vi "Uart log catch.vi"() -> (10 "Key word 2":i32)   [LabVIEW 2023]
uses:
  <vilib>/Instr/_visa.llb/VISA Configure Serial Port (Instr).vi
  <vilib>/Utility/file.llb/Write Delimited Spreadsheet (string).vi
panel:
  in  "Combo Box 3":string(combo)="mfc"
  in  "Combo Box 2":string(combo)="nu1651"
  in  "search string":string="mfc_auto_test_work: g_auto_test_step = 0x"
  in  "Combo Box":string(combo)="mfc_auto_test_work"
  in  "Clear":bool
  in  "VISA resource name":refnum<visa-resource-name>="COM15"
  out "Key word log 2":string
  out "Key word log 1":string
  out "Full log":string
  in  "stop":bool
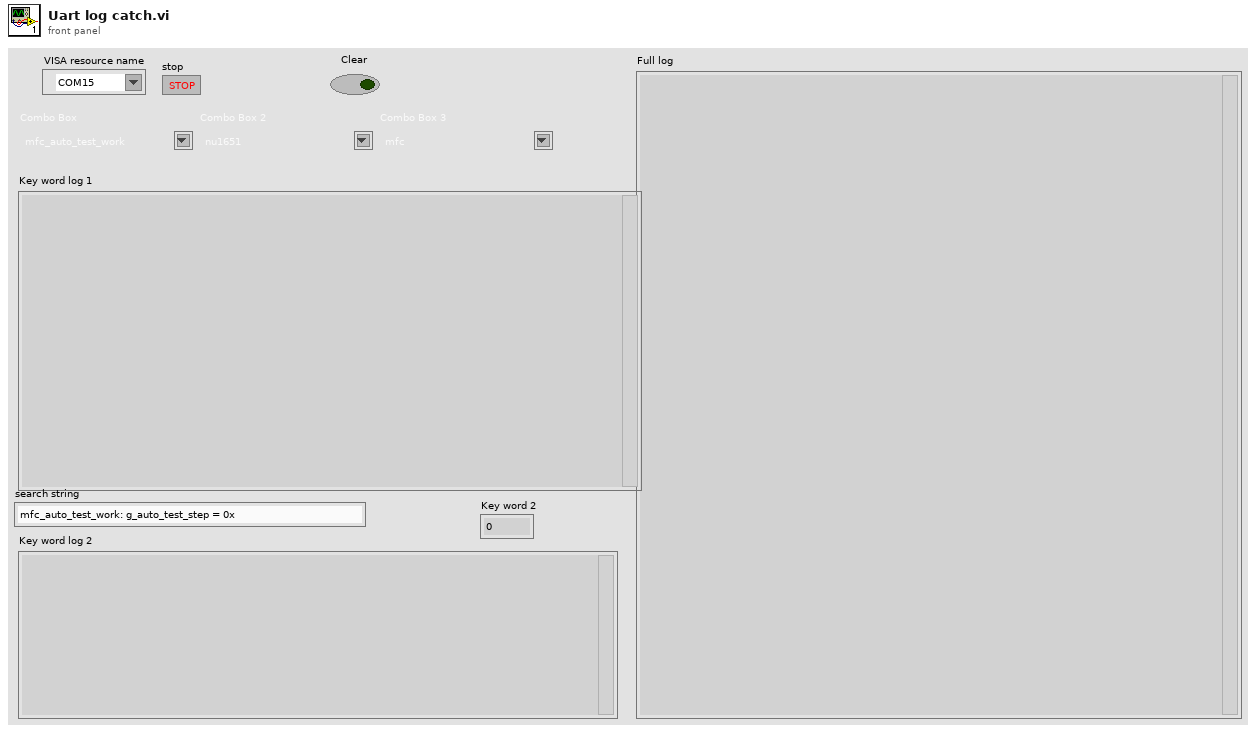
[diagram p1: front panel]
types:
  T1 = enum16{"open", "replace", "create", "open or create", "replace or create", "replace or create with confirmation"}
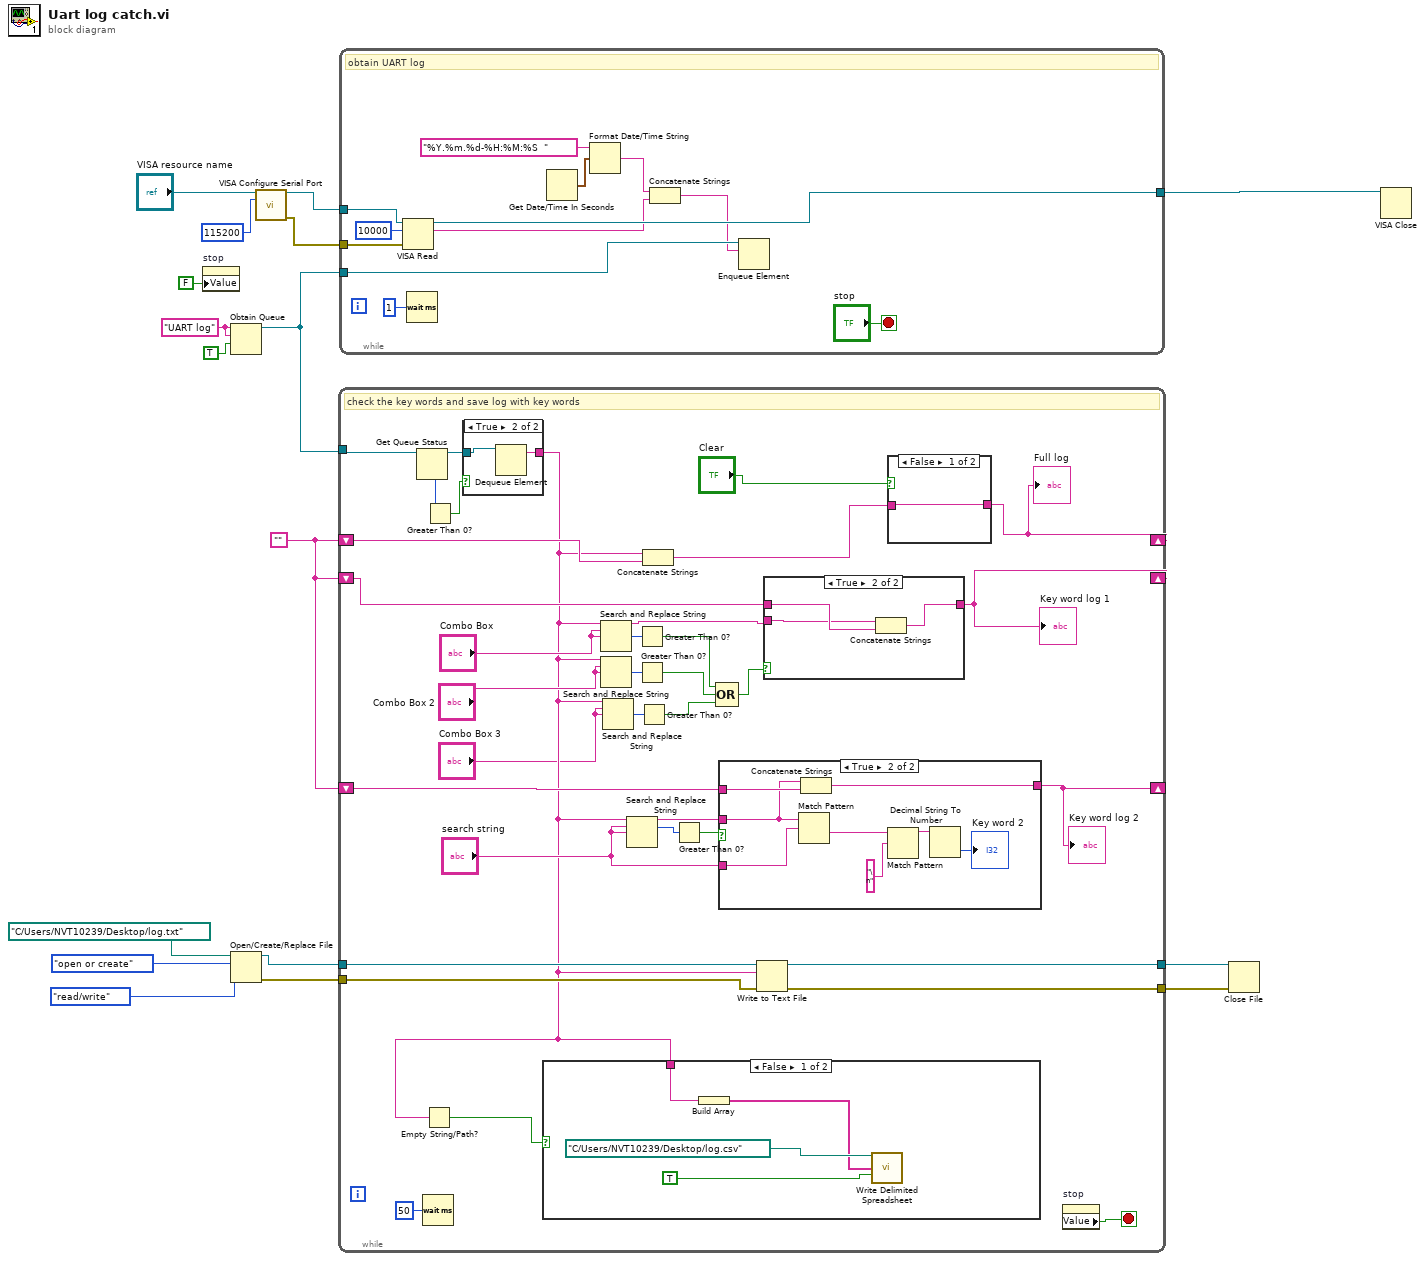
[diagram p0: block diagram]
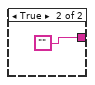
[diagram p3: hidden frame]
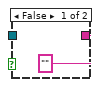
[diagram p6: hidden frame]
diagram:
  w10 = ""
  w16 = "UART log" ("name (unnamed)")
  n1 = property on="stop" class="Bool (strict)"("Value"=FALSE ("stop")) -> ()  [unwired: 2 in, 2 out]
  n2 = Obtain Queue(name (unnamed)=w16, element data type=w16, create if not found? (T)=TRUE) -> (queue out=w8:refnum<queue>)  [unwired: 2 in, 2 out]
  n3 = Open/Create/Replace File(file path (use dialog)=path "C:/Users/NVT10239/Desktop/log.txt", operation (0:open)=T1."open or create", access (0:read/write)=enum16{"read/write", "read-only", "write-only"}."read/write") -> (refnum out=w4:refnum<file>, error out=w3:errorcluster)  [unwired: 3 in, 1 out]
  n4 = call-poly "VISA Configure Serial Port"("VISA resource name"="VISA resource name", "baud rate (9600)"=u32 115200) -> ("VISA resource name out"=w13:refnum<visa-resource-name>, "error out"=w14:errorcluster)  [unwired: 12 in]
  n5 = while {
    tunnel: w8 -> [w37]
    shift-right: [w35] -> _
    shift-left: w10 -> [w48]
    shift-right: [w39] -> _
    shift-left: w10 -> [w44]
    shift-right: [w38] -> _
    shift-left: w10 -> [w40]
    tunnel: w4 -> [w33]
    tunnel: w3 -> [w32]
    tunnel: [w31] -> w2
    tunnel: [w30] -> w1
    stop <- w49 stop-if-true
    # "check the key words and save log with key words"
    n6 = Get Queue Status(queue=w37) -> (queue out=w52:refnum<queue>, # elements in queue=w46:i32)  [unwired: 2 in, 6 out]
    n7 = Wait (ms)(milliseconds to wait=u32 50) -> ()  [unwired: 1 out]
    n8 = Greater Than 0?(x=w46) -> (x > 0?=w51:bool)
    n9 = case shown="True" w51 {
      tunnel: w52 -> [_ w74]
      tunnel: ["" w73] -> w23
      frame False {
      }
      frame True {
        n10 = Dequeue Element(queue=w74) -> (element=w73:string)  [unwired: 2 in, 3 out]
      }
    }
    n11 = Empty String/Path?(string/path=w23) -> (empty?=w29:bool)
    n12 = case shown="False" w29 {
      tunnel: w23 -> [w55 _]
      frame False {
        n13 = Build Array "Build Array"(w55) -> (w54:string[])
        n14 = call-poly <vilib>:"Write Delimited Spreadsheet.vi"("file path (dialog if empty)"=path "C:/Users/NVT10239/Desktop/log.csv" ("file path (use dialog)"), "1D data"=w54, "append to file? (new file:F)"=TRUE) -> ()  [unwired: 11 in, 2 out]
      }
      frame True {
      }
    }
    n15 = Search and Replace String(input string=w23, search string="Combo Box", replace string="Combo Box") -> (result string=w45:string, number of replacements=w47:i32)  [unwired: 5 in, 2 out]
    n16 = Search and Replace String(input string=w23, search string="Combo Box 2", replace string="Combo Box 2") -> (number of replacements=w26:i32)  [unwired: 5 in, 3 out]
    n17 = Search and Replace String(input string=w23, search string="Combo Box 3", replace string="Combo Box 3") -> (number of replacements=w24:i32)  [unwired: 5 in, 3 out]
    n18 = Search and Replace String(input string=w23, search string="search string", replace string="search string") -> (result string=w41:string, number of replacements=w43:i32)  [unwired: 5 in, 2 out]
    n19 = Greater Than 0?(x=w47) -> (x > 0?=w20:bool)
    n20 = Greater Than 0?(x=w26) -> (x > 0?=w19:bool)
    n21 = Greater Than 0?(x=w24) -> (x > 0?=w18:bool)
    n22 = Concatenate Strings "Concatenate Strings"(w23, w48) -> (w36:string)
    n23 = Greater Than 0?(x=w43) -> (x > 0?=w42:bool)
    n24 = Compound Arithmetic op=OR(w20, w19, w18) -> (w21:bool)
    n25 = case shown="True" w42 {
      tunnel: [w59 w67] -> w38
      tunnel: w41 -> [_ w60]
      tunnel: w40 -> [w59 w62]
      tunnel: "search string" -> [_ w61]
      frame False {
      }
      frame True {
        n26 = Match Pattern(string=w60, regular expression=w61) -> (after substring=w65:string)  [unwired: 1 in, 3 out]
        n27 = Concatenate Strings(w60, w62) -> (w67:string)
        n28 = Match Pattern(string=w65, regular expression="\n") -> (before substring=w66:string)  [unwired: 1 in, 3 out]
        n29 = Decimal String To Number(string=w66) -> (number=→"Key word 2":i32)  [unwired: 2 in, 1 out]
      }
    }
    "Key word log 2" <- w38
    n30 = Write to Text File(file (use dialog)=w33, text=w23, error in=w32) -> (refnum out=w31:refnum<file>, error out=w30:errorcluster)  [unwired: 1 in, 1 out]
    n31 = case shown="True" w21 {
      tunnel: w44 -> [w68 w71]
      tunnel: [w68 w70] -> w39
      tunnel: w45 -> [_ w69]
      frame False {
      }
      frame True {
        n32 = Concatenate Strings(w69, w71) -> (w70:string)
      }
    }
    "Key word log 1" <- w39
    n33 = case shown="False" "Clear" {
      tunnel: w36 -> [w57 _]
      tunnel: [w57 ""] -> w35
      frame False {
      }
      frame True {
      }
    }
    "Full log" <- w35
    n34 = property on="stop" class="Bool (strict)"() -> ("Value"=w49:bool)  [unwired: 2 in, 2 out]
  }
  n35 = while {
    tunnel: w8 -> [w86]
    tunnel: w14 -> [w85]
    tunnel: w13 -> [w84]
    tunnel: [w80] -> w11
    stop <- "stop" stop-if-true
    # "obtain UART log"
    n36 = VISA Read(VISA resource name=w84, byte count=u32 10000, error in (no error)=w85) -> (VISA resource name out=w80:refnum<visa-resource-name>, read buffer=w79:string)  [unwired: 2 out]
    n37 = Wait (ms)(milliseconds to wait=u32 1) -> ()  [unwired: 1 out]
    n38 = Get Date/Time In Seconds() -> (seconds since 1Jan1904=w78:timestamp)
    n39 = Format Date/Time String(time format string (%c)="%Y.%m.%d-%H:%M:%S  ", seconds (now)=w78) -> (date/time string=w76:string)  [unwired: 1 in]
    n40 = Concatenate Strings(w76, w79) -> (w75:string)
    n41 = Enqueue Element(queue=w86, element=w75) -> ()  [unwired: 2 in, 3 out]
  }
  n42 = Close File(refnum=w2, error in=w1) -> ()  [unwired: 2 out]
  n43 = VISA Close(VISA resource name=w11) -> ()  [unwired: 1 in, 1 out]
